vi "Join Packets.vi"(3 "error in (no error)":errorcluster, 5 "Packets":string[](array[string])) -> (0 "error out":errorcluster, 2 "Response":string)   [LabVIEW 2018, in "Zaber A Series.lvlib"]
doc: "This VI combines the packets of a multi-packet message into a single long message, and validates any checksums present on the input packets. \n\nMulti-packet messages can occur in some responses from Zaber controllers with four or more axes. They are indicated by the presence of '\\' in the initial packet and \"cont\" in the continuation packets.\n\nThis VI expects the input array to contain ALL and ONLY the packets comprising one response from one device, and that they are in the correct order. The input packets may have the original line endings still present, and may have checksums. The output packet will not have a line ending nor a checksum.\n\nChecksum errors and some message sequence errors are checked for. If an error is detected or if the error input is set to an error condition, the output response will be an empty string.\n\nNote that if you broadcast a command or quickly send commands to multiple devices, it is possible for a reply from device to be interleaved between the packets of a reply from another device. This use case is not supported; this library does not provide the level of message correlation needed to handle it."
uses:
  Zaber A Series.lvlib
panel:
  # "(c) 2017-2020 Zaber Technologies.  ALL RIGHTS RESERVED."
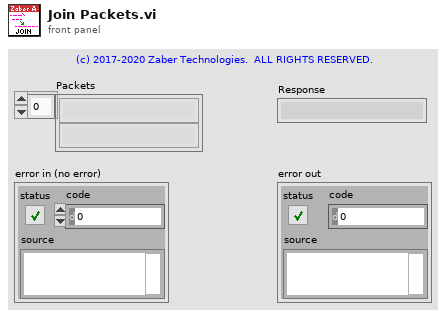
[diagram p1: front panel]
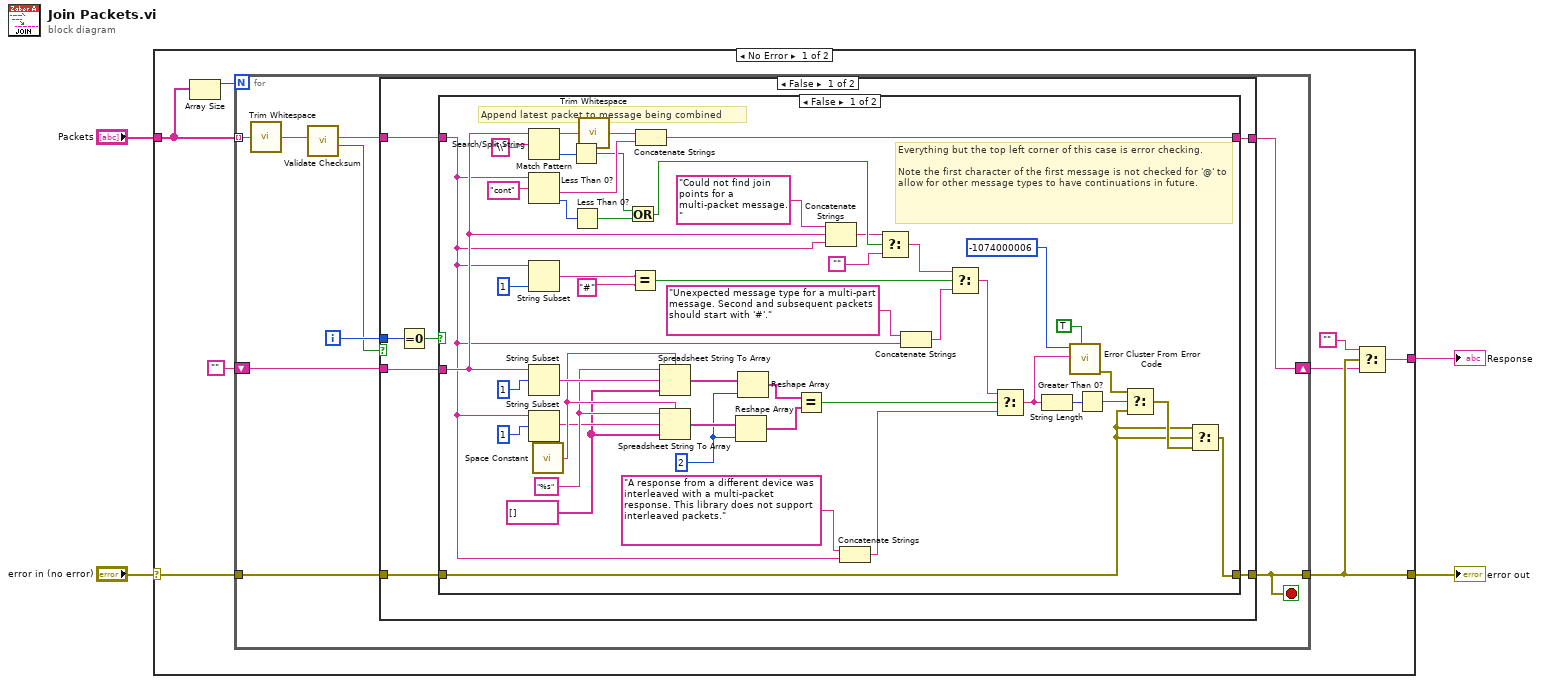
[diagram p0: block diagram]
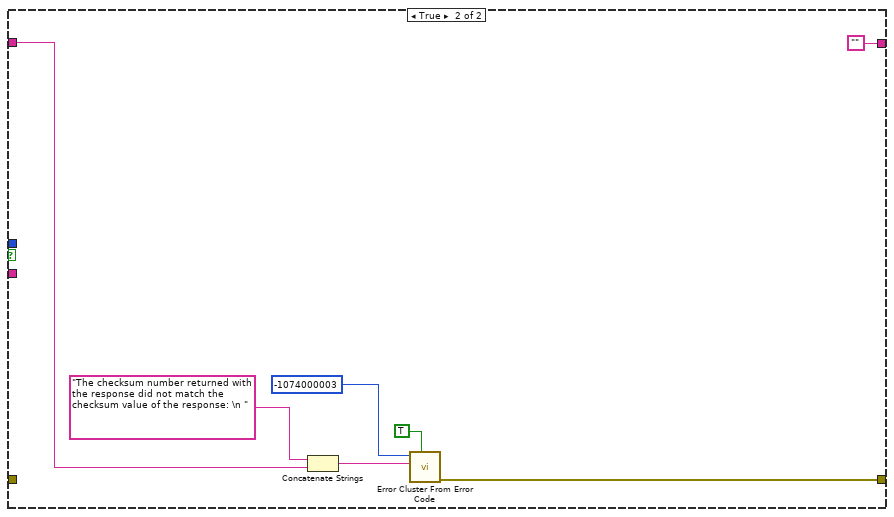
[diagram p3: hidden frame]
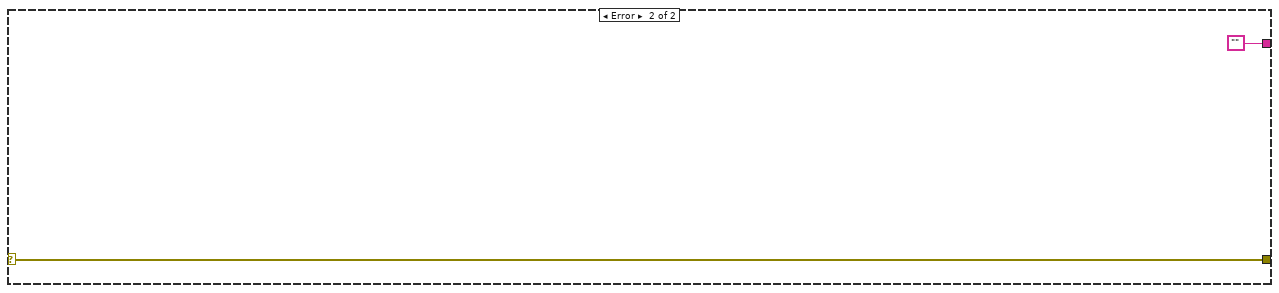
[diagram p4: hidden frame]
diagram:
  n1 = case shown="No Error" "error in (no error)" {
    selector: "error in (no error)" -> [w9 w87]
    tunnel: [w8 w87] -> w3
    tunnel: "Packets" -> [w11 _]
    tunnel: [w7 ""] -> w2
    frame No Error {
      n2 = Array Size(array=w11) -> (size(s)=w12:i32)
      n3 = for {
        N: w12 -> [_]
        tunnel: w11 -> [w17] mode=indexing
        shift-right: [w21] -> w5
        shift-left: "" -> [w20]
        tunnel: w9 -> [w18]
        tunnel: [w13] -> w8
        i -> [w19]
        stop <- w13 stop-if-true
        n4 = call <vilib>:"Trim Whitespace.vi"("string"=w17) -> ("trimmed string"=w16:string)  [unwired: 1 in]
        n5 = call "Validate Checksum.vi"("Response"=w16) -> ("Invalid Checksum?"=w14:bool, "Remaining Response"=w15:string)  [unwired: 9 in]
        n6 = case shown="False" w14 {
          tunnel: [w28 ""] -> w21
          tunnel: w20 -> [w27 _]
          tunnel: w19 -> [w26 _]
          tunnel: [w24 w81] -> w13
          tunnel: w18 -> [w23 _]
          tunnel: w15 -> [w22 w80]
          frame False {
            n7 = Equal To 0?(x=w26) -> (x = 0?=w25:bool)
            n8 = case shown="False" w25 {
              tunnel: [w76 w78] -> w28
              tunnel: w27 -> [w46 _]
              tunnel: w22 -> [w29 w78]
              tunnel: [w43 w77] -> w24
              tunnel: w23 -> [w30 w77]
              frame False {
                w60 = 2 ("dimension size")
                w63 = string[] []
                w65 = "%s" ("format string")
                # "Everything but the top left corner of this case is error checking.\n\nNote the first character of the first message is not checked for '@' to allow for other message types to have continuations in future."
                # "Append latest packet to message being combined"
                n9 = Search/Split String(string=w46, search string/char (-)="\\") -> (substring before match=w45:string, offset of match=w72:i32)  [unwired: 1 in, 1 out]
                n10 = Match Pattern(string=w29, regular expression="cont") -> (after substring=w73:string, offset past match=w71:i32)  [unwired: 1 in, 2 out]
                n11 = String Subset(string=w29, length (rest)=1 ("length (rest)")) -> (substring=w53:string)  [unwired: 1 in]
                n12 = String Subset(string=w46, offset (0)=1 ("length (rest)")) -> (substring=w67:string)  [unwired: 1 in]
                n13 = String Subset(string=w29, offset (0)=1 ("length (rest)")) -> (substring=w64:string)  [unwired: 1 in]
                n14 = call <vilib>:"Space Constant.vi"() -> ("String"=w66:string)
                n15 = Less Than 0?(x=w72) -> (x < 0?=w49:bool)
                n16 = Less Than 0?(x=w71) -> (x < 0?=w48:bool)
                n17 = call <vilib>:"Trim Whitespace.vi"("string"=w45) -> ("trimmed string"=w44:string)  [unwired: 1 in]
                n18 = Or(x=w49, y=w48) -> (x .or. y?=w39:bool)
                n19 = Equal?(x=w53, y="#") -> (x = y?=w51:bool)
                n20 = Concatenate Strings(w44, w73) -> (w76:string)
                n21 = Spreadsheet String To Array(delimiter (Tab)=w66, format string=w65, spreadsheet string=w67, array type (2D Dbl)=w63) -> (array=w62:string[])
                n22 = Spreadsheet String To Array(delimiter (Tab)=w66, format string=w65, spreadsheet string=w64, array type (2D Dbl)=w63) -> (array=w61:string[])
                n23 = Reshape Array(w61, w60) -> (w58:string[])
                n24 = Reshape Array(w62, w60) -> (w59:string[])
                n25 = Equal?(x=w59, y=w58) -> (x = y?=w57:bool)
                n26 = Concatenate Strings("Could not find join points for a multi-packet message." ("error message (\"\")"), w46, w29) -> (w38:string)
                n27 = Concatenate Strings("A response from a different device was interleaved with a multi-packet response. This library does not support interleaved packets." ("error message (\"\")"), w29) -> (w42:string)
                n28 = Select(t=w38, s=w39, f="") -> (s? t:f=w37:string)
                n29 = Concatenate Strings("Unexpected message type for a multi-part message. Second and subsequent packets should start with '#'." ("error message (\"\")"), w29) -> (w41:string)
                n30 = Select(t=w37, s=w51, f=w41) -> (s? t:f=w50:string)
                n31 = Select(t=w50, s=w57, f=w42) -> (s? t:f=w35:string)
                n32 = String Length(string=w35) -> (length=w34:i32)
                n33 = call <vilib>:"Error Cluster From Error Code.vi"("show call chain? (False)"=TRUE, "error message (\"\")"=w35, "error code (0)"=-1074000006) -> ("error out"=w32:errorcluster)  [unwired: 6 in]
                n34 = Greater Than 0?(x=w34) -> (x > 0?=w33:bool)
                n35 = Select(t=w32, s=w33, f=w30) -> (s? t:f=w31:errorcluster)
                n36 = Select(t=w30, s=w30, f=w31) -> (s? t:f=w43:errorcluster)
              }
              frame True {
                # "Just store the first packet as\nthe start of the combined \nmessage."
              }
            }
          }
          frame True {
            n37 = Concatenate Strings("The checksum number returned with the response did not match the checksum value of the response: \n " ("error message (\"\")"), w80) -> (w84:string)
            n38 = call <vilib>:"Error Cluster From Error Code.vi"("show call chain? (False)"=TRUE, "error message (\"\")"=w84, "error code (0)"=-1074000003) -> ("error out"=w81:errorcluster)  [unwired: 6 in]
          }
        }
      }
      n39 = Select(t="", s=w8, f=w5) -> (s? t:f=w7:string)
    }
    frame Error {
    }
  }
  "error out" <- w3
  "Response" <- w2
